vi "Get Modified Timestamp.vi"(8 "error in (no error)":errorcluster, 10 "RemoteFileName":string, 11 "FTP in":refnum<class "FTP.lvclass">) -> (0 "error out":errorcluster, 2 "Modified Timestamp":timestamp, 3 "FTP out":refnum<class "FTP.lvclass">)   [LabVIEW 2020, in "FTP.lvlib" / "FTP.lvclass"]
doc: "This vi will return the modified time stamp for the file specified by the \"RemoteFileName\" parameter. Not all FTP servers will respond to this command. Only FTP servers with the MDTM feature available will respond appropriately."
uses:
  FTP.lvclass
  FTP.lvclass/FTP.ctl
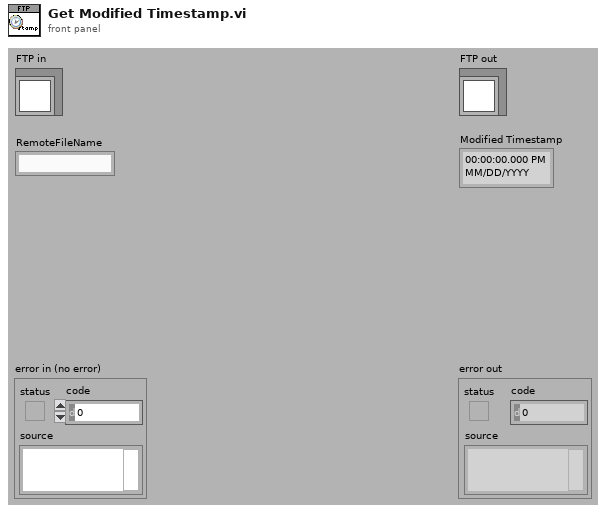
[diagram p1: front panel]
types:
  T1 = typedef "FTP.lvlib/FTP.lvclass/Dir-File Info.ctl" = cluster{"Name":string, "Modify Timestamp":timestamp, "Dir-File Type":T2, "Unique Id":string, "Permissions":string, "Unix Mode":u16, "Owner":string, "Group":string, "FileSize":i64}
  T2 = typedef "FTP.lvlib/FTP.lvclass/Dir-File Type.ctl" = enum16{"File", "Listed Directory", "Parent Directory", "Directory", "Unknown"}
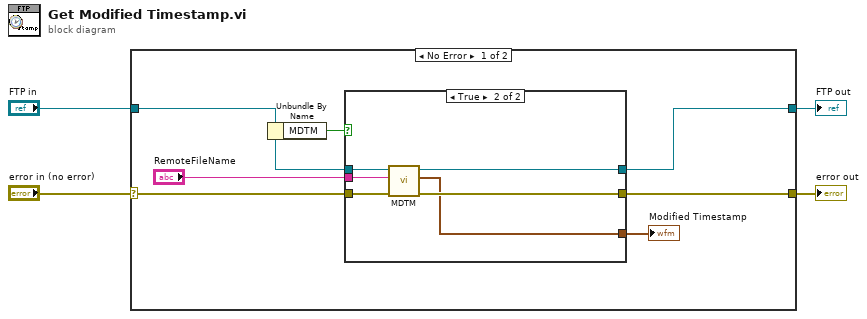
[diagram p0: block diagram]
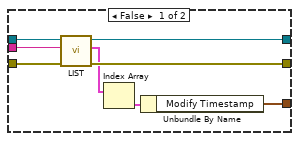
[diagram p2: hidden frame]
diagram:
  n1 = case shown="No Error" "error in (no error)" {
    selector: "error in (no error)" -> [w11 w27]
    tunnel: [w9 w27] -> w3
    tunnel: [w10 w26] -> w1
    tunnel: "FTP in" -> [w6 w26]
    frame No Error {
      n2 = Unbundle By Name(w6) -> ("MDTM"=w5:bool)
      n3 = case shown="True" w5 {
        tunnel: w11 -> [w19 w25]
        tunnel: [w16 w24] -> w10
        tunnel: [w15 w23] -> w9
        tunnel: "RemoteFileName" -> [w17 w22]
        tunnel: [w12 w21] -> w7
        tunnel: w6 -> [w18 w20]
        frame False {
          n4 = call "LIST.vi"("error in (no error)"=w19, "Remote File"=w17, "FTP in"=w18) -> ("error out"=w15:errorcluster, "Dir-File Info Array"=w14:T1[], "FTP out"=w16:refnum<class "FTP.lvclass">)  [unwired: 6 in]
          n5 = Index Array(array=w14) -> (element=w13:T1)  [unwired: 1 in]
          n6 = Unbundle By Name(w13) -> ("Modify Timestamp"=w12:timestamp)
        }
        frame True {
          n7 = call "MDTM.vi"("error in (no error)"=w25, "RemoteFileName"=w22, "FTP in"=w20) -> ("error out"=w23:errorcluster, "Modified Timestamp"=w21:timestamp, "FTP out"=w24:refnum<class "FTP.lvclass">)  [unwired: 6 in]
        }
      }
      "Modified Timestamp" <- w7
    }
    frame Error {
    }
  }
  "error out" <- w3
  "FTP out" <- w1
